vi "WSVCAP SHL Host TL I2C Write - Multiple Device - Common Data.vi"(0 "Sub Address":u8=20 format="%.0x", 3 "FPGA":T1, 5 "Data Out [U8]":u8=20 format="%.0x", 11 "error in":errorcluster, 12 "Log (T)":bool=TRUE, 13 "DUT Mask Array (All)":bool[](array[boolean])=[TRUE, TRUE, TRUE, TRUE, TRUE, TRUE, TRUE, TRUE, TRUE, TRUE, TRUE, TRUE, TRUE, TRUE, TRUE, TRUE, TRUE, TRUE, TRUE, TRUE, TRUE, TRUE, TRUE, TRUE, TRUE, TRUE, TRUE, TRUE, TRUE, TRUE, TRUE, TRUE, TRUE, TRUE, TRUE, TRUE, TRUE, TRUE, TRUE, TRUE, TRUE, TRUE, TRUE, TRUE, TRUE, TRUE, TRUE, TRUE, TRUE, TRUE, TRUE, TRUE, TRUE, TRUE, TRUE, TRUE, TRUE, TRUE, TRUE, TRUE, TRUE, TRUE, TRUE, TRUE], 14 "DUT Mask Mode (All)":T2=enum."All") -> (15 "error out":errorcluster)   [LabVIEW 2017]
uses:
  Type Defs/WSVCAP SHL I2C DUT Mask Mode Enum.ctl
  Type Defs/WSVCAP SHL FPGA Enum.ctl
panel:
  out "Socket Mask [U64]":u64 format="%016x"
  out "C1 Data Out":u8[](array[numeric]) format="%.0x"
  # "DUT 01"
  # "DUT 02"
  # "DUT 03"
  # "DUT 04"
  # "DUT 05"
  # "DUT 06"
  # "DUT 07"
  # "DUT 08"
  # "DUT 09"
  # "DUT 10"
  # "DUT 11"
  # "DUT 12"
  # "DUT 13"
  # "DUT 14"
  # "DUT 15"
  # "DUT 16"
  # "DUT 17"
  # "DUT 18"
  # "DUT 19"
  # "DUT 20"
  # "DUT 21"
  # "DUT 22"
  # "DUT 23"
  # "DUT 24"
  # "DUT 25"
  # "DUT 26"
  # "DUT 27"
  # "DUT 28"
  # "DUT 29"
  # "DUT 30"
  # "DUT 31"
  # "DUT 32"
  # "DUT 33"
  # "DUT 34"
  # "DUT 35"
  # "DUT 36"
  # "DUT 37"
  # "DUT 38"
  # "DUT 39"
  # "DUT 40"
  # "DUT 41"
  # "DUT 42"
  # "DUT 43"
  # "DUT 44"
  # "DUT 45"
  # "DUT 46"
  # "DUT 47"
  # "DUT 48"
  # "DUT 49"
  # "DUT 50"
  # "DUT 51"
  # "DUT 52"
  # "DUT 53"
  # "DUT 54"
  # "DUT 55"
  # "DUT 56"
  # "DUT 57"
  # "DUT 58"
  # "DUT 59"
  # "DUT 60"
  # "DUT 61"
  # "DUT 62"
  # "DUT 63"
  # "DUT 64"
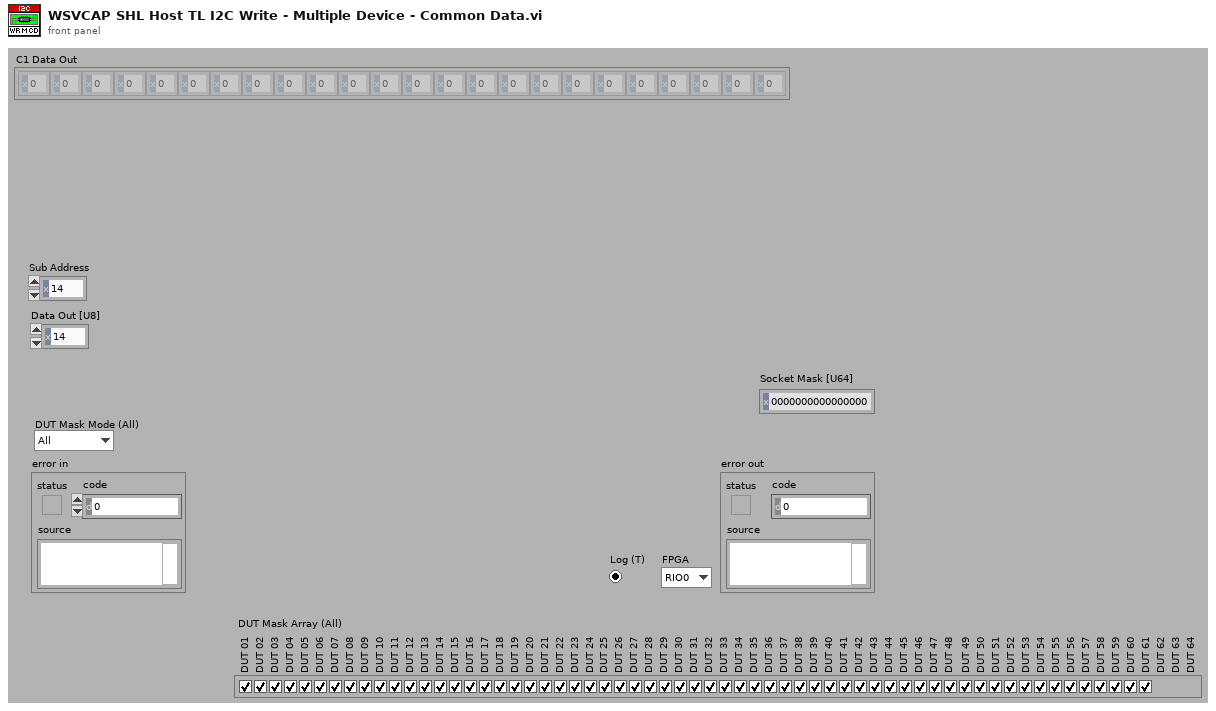
[diagram p1: front panel]
types:
  T1 = typedef "WSVCAP SHL FPGA Enum.ctl" = enum16{"RIO0", "RIO1"}
  T2 = typedef "WSVCAP SHL I2C DUT Mask Mode Enum.ctl" = enum16{"Custom", "All"}
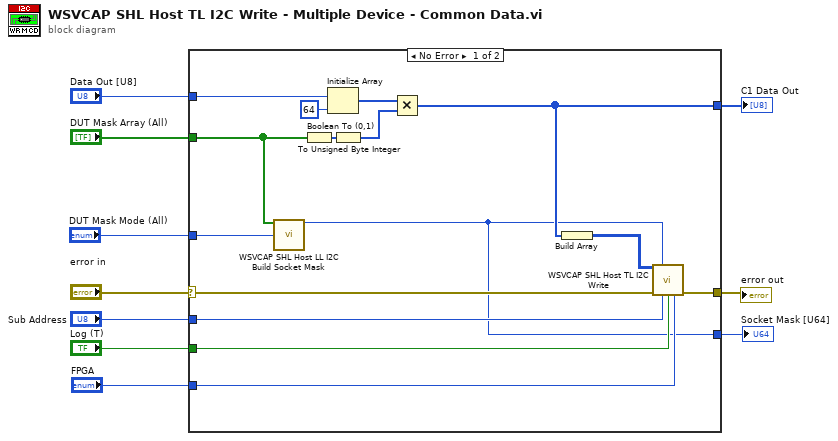
[diagram p0: block diagram]
diagram:
  n1 = case shown="No Error" "error in" {
    selector: "error in" -> [w19 w26]
    tunnel: [w25 w26] -> w10
    tunnel: "Sub Address" -> [w17 _]
    tunnel: "Data Out [U8]" -> [w22 _]
    tunnel: [w20 _] -> w6
    tunnel: [w12 _] -> w5
    tunnel: "DUT Mask Array (All)" -> [w16 _]
    tunnel: "Log (T)" -> [w18 _]
    tunnel: "DUT Mask Mode (All)" -> [w15 _]
    tunnel: "FPGA" -> [w14 _]
    frame No Error {
      n2 = call "WSVCAP SHL Host LL I2C Build Socket Mask.vi"("DUT Mask Array"=w16, "DUT Mask Mode (Custom)"=w15) -> ("Socket Mask Set [U64]"=w12:u64)  [unwired: 13 in]
      n3 = Boolean To (0,1)(Boolean=w16) -> (0, 1=w23:i16[])
      n4 = Initialize Array(w22, 64 ("dimension size")) -> (w13:u8[])
      n5 = To Unsigned Byte Integer(number=w23) -> (unsigned 8bit integer=w11:u8[])
      n6 = Multiply(x=w13, y=w11) -> (x*y=w20:u8[])
      n7 = Build Array(w20) -> (w24:u8[][])
      n8 = call "WSVCAP SHL Host TL I2C Write.vi"("C Data Out"=w24, "Socket Mask [U64]"=w12, "error in"=w19, "Sub Address"=w17, "Log (T)"=w18, "FPGA"=w14) -> ("error out"=w25:errorcluster)  [unwired: 9 in]
    }
    frame Error {
    }
  }
  "error out" <- w10
  "C1 Data Out" <- w6
  "Socket Mask [U64]" <- w5
